vi "WriteToLogFile.vi"(0 "Left thickness":string, 1 "Right thickness":string, 2 "Average thickness":string, 3 "Left residue":string, 4 "Right residue":string, 5 "Target thickness":string, 6 "Deviation":string, 7 "Left in range?":string, 8 "Glass name":string, 9 "Right in range?":string, 10 "Measurement type":string, 11 "Average in range?":string) -> ()   [LabVIEW 2013]
uses:
  Global.vi
  <vilib>/Utility/file.llb/Write To Spreadsheet File (string).vi
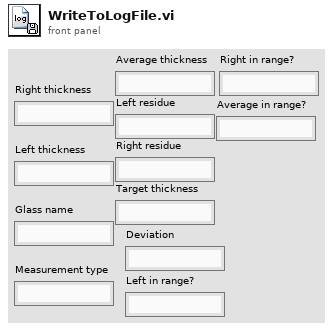
[diagram p1: front panel]
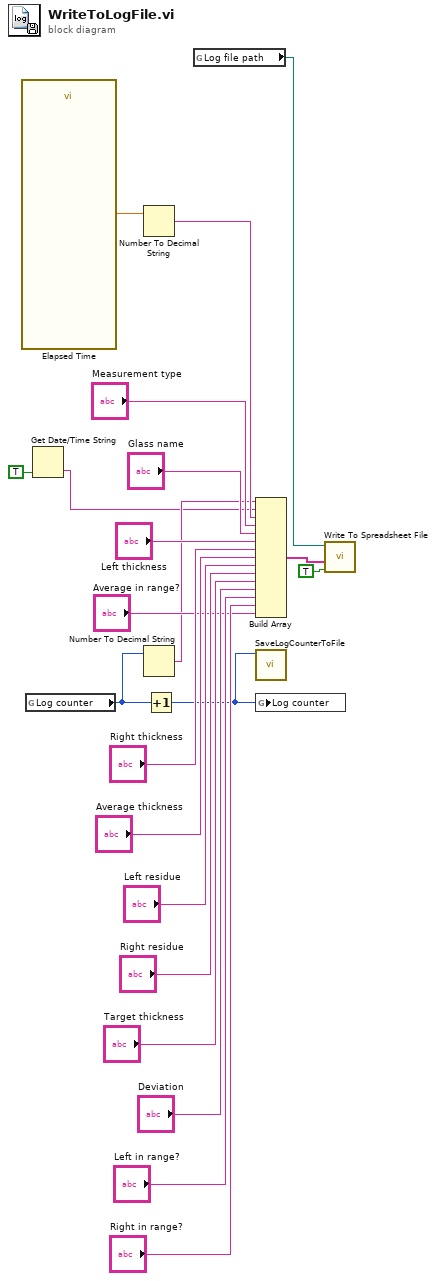
[diagram p0: block diagram]
diagram:
  n1 = call "Elapsed Time"() -> ("Present (s)"=w5:dbl)  [unwired: 12 in, 7 out]
  n2 = global read "Global.vi" "Log counter"() -> (w7:i32)
  n3 = Get Date/Time String(want seconds? (F)=TRUE) -> (time string=w2:string)  [unwired: 2 in, 1 out]
  n4 = Number To Decimal String(number=w5) -> (decimal integer string=w4:string)  [unwired: 1 in]
  n5 = Number To Decimal String(number=w7) -> (decimal integer string=w3:string)  [unwired: 1 in]
  n6 = Increment(x=w7) -> (x+1=w6:i32)
  n7 = global read "Global.vi" "Log file path"() -> (w16:path)
  n8 = Build Array(w3, w2, w4, "Measurement type", "Glass name", "Left thickness", "Right thickness", "Average thickness", "Left residue", "Right residue", "Target thickness", "Deviation", "Left in range?", "Right in range?", "Average in range?") -> (w21:string[])
  n9 = call "SaveLogCounterToFile.vi"("number"=w6) -> ()  [unwired: 11 in]
  n10 = global write "Global.vi" "Log counter"(w6) -> ()
  n11 = call-poly <vilib>:"Write To Spreadsheet File.vi"("append to file? (new file:F)"=TRUE, "1D data"=w21, "file path (dialog if empty)"=w16) -> ()  [unwired: 5 in, 1 out]
